vi "Read Config Unitest.vi"(8 "error in (no error)":errorcluster, 11 "main ref":T1) -> (0 "error out":errorcluster)   [LabVIEW 2025]
uses:
  controls/LAB-IQ UI Data.ctl
  Config file  FGV Unitest enum.ctl
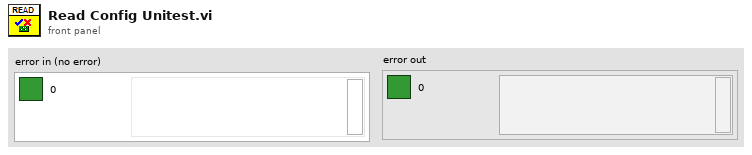
[diagram p1: front panel]
types:
  T1 = typedef "LAB-IQ UI Data.ctl" = cluster{"Main Home Screen":cluster{"GUI":refnum<vi>, "Platform Settings":refnum<vi>, "Configure":refnum<vi>, "Home":refnum<vi>, "EXIT":refnum<vi>, "service 2":refnum<vi>, "MainPage":refnum<vi>, "Analysis":refnum<vi>}, "Platform Settings":cluster{"mm/s  Surge":refnum<vi>, "Update Surge Speed":refnum<vi>, "Drive Error":refnum<vi>, "Disable Axis Jog Soft Limits":refnum<vi>, "mm/s  Sway":refnum<vi>, "Sway and Surge COM Status":refnum<vi>, "Heave COM Status":refnum<vi>, "Enable Platform":refnum<vi>, "Surge Forward Main":refnum<vi>, "Sway Right Main":refnum<vi>, "Sway Left Main":refnum<vi>, "Heave Down Main":refnum<vi>, "Heave Up main":refnum<vi>, "Update Sway Speed":refnum<vi>, "Update Heave Speed":refnum<vi>, "mm/s Heave":refnum<vi>, "mm/sec":refnum<vi>, "mm":refnum<vi>, "Surge Backward Main":refnum<vi>}, "Analysis Screen":cluster{"Analysis Home":refnum<vi>, "Surface Analysis":refnum<vi>, "Imaging":refnum<vi>, "Image Analysis":refnum<vi>, "Post Analysis":refnum<vi>}, "Config Screen":cluster{"Select Load Head":refnum<vi>, "Notes :":refnum<vi>, "FILE":refnum<vi>, "Sample ID :":refnum<vi>, "Operator ID :":refnum<vi>, "Operator Name :":refnum<vi>, "Auto":refnum<vi>}, "Motion Module":cluster{"zNL":refnum<vi>, "NL disp":refnum<vi>, "Rotary Tab":refnum<vi>, "Motion Direction:  3":refnum<vi>, "E.Velocity 2":refnum<vi>, "e.v/ssr 2":refnum<vi>, "Enter Fixed E.Velocity 2":refnum<vi>, "Enter Final SRR 2":refnum<vi>, "Enter initial SRR 2":refnum<vi>, "Enter Fixed SRR 2":refnum<vi>, "Enter the Final E.Velocity (m/s) 2":refnum<vi>, "Enter initial E.Velocity (m/s) 2":refnum<vi>, "Final Speed (RPM) 3":refnum<vi>, "Initial Speed (RPM) 2":refnum<vi>, "Enter the Final Velocity (m/s) 3":refnum<vi>, "Enter initial Velocity (m/s)  3":refnum<vi>, "Ramp Up 2":refnum<vi>, "TEST SELECTION":refnum<vi>, "SPEED SELECTION : ":refnum<vi>, "Angular Oscillation Set":refnum<vi>, "Traction":refnum<vi>, "Step Speed":refnum<vi>, "StepTable For Load-Speed":refnum<vi>, "StepTable For Speed":refnum<vi>, "Surge Forward MM":refnum<vi>, "Surge Backward MM":refnum<vi>, "M3 Image":refnum<vi>, "String 39":refnum<vi>, "Sway Left MM":refnum<vi>, "Sway Right MM":refnum<vi>, "Disable Axis Jog Soft Limits":refnum<vi>, "mm":refnum<vi>, "Heave Down MM":refnum<vi>, "Heave Up MM":refnum<vi>, "Wear Track Diameter (mm)":refnum<vi>, "Set WTD":refnum<vi>, "HomeScratch":refnum<vi>, "HomeRot":refnum<vi>, "PlaceModule":refnum<vi>, "Enter the Angle (Deg)":refnum<vi>, "Enter the Frequency (Hz)":refnum<vi>, "Motion Mode:":refnum<vi>, "LR Sway":refnum<vi>, "Rot Hor":refnum<vi>, "Scratch":refnum<vi>, "LR Cam":refnum<vi>, "MMBack":refnum<vi>, "MMNext":refnum<vi>, "Rot Ver":refnum<vi>, "Rotary Module Selection":refnum<vi>, "calculate rotary":refnum<vi>, "SPEED SELECTION : rotary":refnum<vi>, "Import 2":refnum<vi>, "Save 2":refnum<vi>, "File Path :  2":refnum<vi>, "String 45":refnum<vi>, "StepTable For Speed 3":refnum<vi>, "Enter the Speed(mm/sec)":refnum<vi>, "Enter the Speed(RPM)":refnum<vi>, "Enter Scratch Speed (mm/s):":refnum<vi>, "SwaySpeed Set":refnum<vi>, "Scartch Offset":refnum<vi>, "Motion type:":refnum<vi>, "HomeScratch 2":refnum<vi>, "Enter Scratch length (mm):":refnum<vi>, "Wear Track Diameter":refnum<vi>, "Rotary Speed Exced":refnum<vi>, "Scratch Mode":refnum<vi>, "No of Scratch":refnum<vi>}, "Environmental control":cluster{"Humidity  Status  3":refnum<vi>, "Low Temp  Status  2":refnum<vi>, "TK4 status 2":refnum<vi>, "Stage Temperature":refnum<vi>, "Sample Temperature":refnum<vi>, "Humidity (Amb)":refnum<vi>, "Clear List":refnum<vi>, "Add to list":refnum<vi>, "Wear":refnum<vi>, "Vibration":refnum<vi>, "Humidity (Chamber)":refnum<vi>, "Temperature (Chamber)":refnum<vi>, "ECR ":refnum<vi>, "Temperature (Amb)":refnum<vi>, "Microphone":refnum<vi>, "Acoustic Emission 3":refnum<vi>, "SNext":refnum<vi>, "APBack":refnum<vi>, "Enter the Temperature (°C):":refnum<vi>, "Enter the Stage \nTemperature (°C):":refnum<vi>, "Enter the Humidity (%Rh):":refnum<vi>, "Low Temp":refnum<vi>, "High Temp":refnum<vi>, "Humidity":refnum<vi>, "Sensors Picked":refnum<vi>}, "About Screen":cluster{"Password":refnum<vi>, "Home Service":refnum<vi>, "Advanced Setting":refnum<vi>, "About Tab":refnum<vi>, "ECR Port:":refnum<vi>, "Ramp Port:":refnum<vi>, "Installation/Replacement completed":refnum<vi>, "Loahead":refnum<vi>, "Heave and Surge COM Port:":refnum<vi>, "Sway COM Port:":refnum<vi>, "Temp Modbus:":refnum<vi>, "Humidity Port:":refnum<vi>, "Edit Gain Constants":refnum<vi>, "Save Gain Constants":refnum<vi>}, "Main Screen":cluster{"Main Screen Tab":refnum<vi>, "Angle and Frequency":refnum<vi>, "Stroke (mm)":refnum<vi>, "Angle (Deg)":refnum<vi>, "Main Speed Tab":refnum<vi>, "MTM MOTOR DISPLAY":refnum<vi>, "Disc Speed (m/sec)":refnum<vi>, "Ball Speed (m/sec)":refnum<vi>, "Disc Speed (RPM)":refnum<vi>, "Ball Speed (RPM)":refnum<vi>, "SPEED TAB":refnum<vi>, "Speed (m/sec)":refnum<vi>, "Set Speed (m/sec)":refnum<vi>, "Speed (RPM)":refnum<vi>, "Set Speed":refnum<vi>, "Time Tab":refnum<vi>, "Time ( HH:MM:SS ) 2":refnum<vi>, "Test Duration":refnum<vi>, "Test Duration 4":refnum<vi>, "TEST CYCLE":refnum<vi>, "TOTAL CYCLES":refnum<vi>, "Set Load (N)":refnum<vi>, "Temp Tabs":refnum<vi>, "Heater":refnum<vi>, "TK4 status":refnum<vi>, "ChamberTemp":refnum<vi>, "SetTmp":refnum<vi>, "Controller  Status":refnum<vi>, "ChamberTemp 2":refnum<vi>, "SetTmp 2":refnum<vi>, "Controller  Status 2":refnum<vi>, "ChamberTemp 3":refnum<vi>, "SetTmp 3":refnum<vi>, "Cooling":refnum<vi>, "Load Communication":refnum<vi>, "Ambient \nTemperature":refnum<vi>, "HumCOMStatus":refnum<vi>, "Ambient\n Humidity":refnum<vi>, "Freq (Hz)":refnum<vi>, "Load En":refnum<vi>, "NLt":refnum<vi>, "zNL 2":refnum<vi>, "Humidity On":refnum<vi>, "humidity disp":refnum<vi>, "Set Humidity":refnum<vi>, "NL disp 2":refnum<vi>, "Humidity On 2":refnum<vi>, "humidity disp 2":refnum<vi>, "Set Humidity 2":refnum<vi>, "NL disp 3":refnum<vi>, "AppLoadSeq scratch":refnum<vi>, "Stop Scratch":refnum<vi>, "ClrLog":refnum<vi>, "Trip Log":refnum<vi>, "STOP":refnum<vi>, "Start Test":refnum<vi>, "Test status":refnum<vi>, "AR Led":refnum<vi>, "Data":refnum<vi>, "Health":refnum<vi>, "Sway COM Status":refnum<vi>, "Heave COM Status":refnum<vi>, "Grp Tab":refnum<vi>, "Sub Graph":refnum<vi>, "SD (mm)":refnum<vi>, "Siliding distance Reset Graph":refnum<vi>, "SDGp":refnum<vi>, "Humidity Reset Graph":refnum<vi>, "HumrGp":refnum<vi>, "Acoustic Emission (mV)":refnum<vi>, "Aqucostic Reset Graph":refnum<vi>, "gACQUOS":refnum<vi>, "ECR RESET":refnum<vi>, "ECR":refnum<vi>, "Temperature Reset":refnum<vi>, "Acoustic Emission (mV) 2":refnum<vi>, "Aqucostic Reset Graph 2":refnum<vi>, "gACQUOS 2":refnum<vi>, "ECR RESET 2":refnum<vi>, "ECR 2":refnum<vi>, "Temperature Reset 2":refnum<vi>, "Temperature (deg c)":refnum<vi>, "Speed Reset Graph":refnum<vi>, "Speed Tab":refnum<vi>, "MTM DISC  SPEED":refnum<vi>, "MTM BALL SPEED":refnum<vi>, "speed mm/sec":refnum<vi>, "Hymidity":refnum<vi>, "Humidity Disable trip":refnum<vi>, "CoF Trip  2":refnum<vi>, "Depth Trip":refnum<vi>, "Weart Deapth":refnum<vi>, "Depth Reset Graph":refnum<vi>, "Weart":refnum<vi>, "Depthz":refnum<vi>, "Depth (µm)":refnum<vi>, "WearGp":refnum<vi>, "NL Trip 2":refnum<vi>, "Load pid":refnum<vi>, "Load Disable Trip":refnum<vi>, "Load Reset Graph":refnum<vi>, "NL Display 4":refnum<vi>, "Main Chart 3":refnum<vi>, "BACK":refnum<vi>, "Depth Trip 2":refnum<vi>, "COF TRIP ":refnum<vi>, "Friction Force (N)":refnum<vi>, "FF Reset Graph":refnum<vi>, "FF Disable Trip":refnum<vi>, "FF TRIP":refnum<vi>, "COF Disable Trip":refnum<vi>, "COF Reset Graph":refnum<vi>, "Start Test Temp":refnum<vi>, "zFF":refnum<vi>, "Friction Force (N) Graph":refnum<vi>, "Coefficient of Friction":refnum<vi>, "Scratch Start Test":refnum<vi>, "FF Tab":refnum<vi>, "Cyclic Friction Force (N)":refnum<vi>, "CZ FF":refnum<vi>, "Cyclic Friction Force (N) Graph":refnum<vi>, "Cyclic Coefficient of Friction":refnum<vi>, "Cyclic FF TRIP":refnum<vi>, "Cyclic FF Disable Trip":refnum<vi>, "cyclic COF Disable Trip":refnum<vi>, "cyclic COF TRIP":refnum<vi>, "cyclic COF Reset Graph":refnum<vi>, "Cyclic FF Reset Graph":refnum<vi>, "Test Trip":refnum<vi>, "Multi Scratch Pass":refnum<vi>}, "Loading":cluster{"Indentation":refnum<vi>, "Reference Sample":refnum<vi>, "Load Cell Communication Slide":refnum<vi>, "com 3":refnum<vi>, "com":refnum<vi>, "DecaForce COM Status":refnum<vi>, "Update":refnum<vi>, "Clear 3":refnum<vi>, "seq":refnum<vi>, "Stribeck table":refnum<vi>, "Stribeck Table  For loading":refnum<vi>, "Loading Mode":refnum<vi>, "Enter the Final Load (N)":refnum<vi>, "Enter the CoF Trip":refnum<vi>, "Enter the Friction Force Trip":refnum<vi>, "Enter the Normal load Trip":refnum<vi>, "Enter the Load  (N)":refnum<vi>, "KiloForce":refnum<vi>, "DecaForce ":refnum<vi>, "MicroForce":refnum<vi>, "LHBack":refnum<vi>, "LHNext":refnum<vi>, "Enter the Loading Rate (N/min)":refnum<vi>, "Message":refnum<vi>, "Warning 2":refnum<vi>, "SSP 0.75":refnum<vi>, "SSP 0.5":refnum<vi>, "SSP 0.3":refnum<vi>, "Warning":refnum<vi>, "gui GIF":refnum<vi>, "Communication is established":refnum<vi>, "AppLoad 4":refnum<vi>, "Multipoint":refnum<vi>, "Load Selection":refnum<vi>}, "PID":cluster{"Ramp MulFac":refnum<vi>, "pulses LoadDiffRamp(2..10)":refnum<vi>, "PulseControlRamp(diff<=3N)":refnum<vi>, "SetLoadDeadband(%) Load(0-10N)":refnum<vi>, "PID gains out delay (microForce)":refnum<vi>, "Ramp":refnum<vi>, "Gain 2":refnum<vi>, "pulses LoadDiff(2..10)":refnum<vi>, "pulses LoadDiff(11..50)":refnum<vi>, "PulseControl(diff<=3N)":refnum<vi>, "SetLoadDeadband(%)  2":refnum<vi>, "Dummy Run":refnum<vi>, "Vertical load (N)":refnum<vi>, "AutoTune":refnum<vi>, "Offset 3 ":refnum<vi>, "apply load":refnum<vi>, "Offset  3":refnum<vi>, "apply load 2":refnum<vi>, "Enter ByPass Load":refnum<vi>, "reinit 3":refnum<vi>, "output range delay":refnum<vi>, "PID gains out delay":refnum<vi>, "Bypass Load":refnum<vi>, "pulsesSent":refnum<vi>, "pulses ":refnum<vi>, "actpid":refnum<vi>, "gFF Rot":refnum<vi>, "pulses LoadDiff(21..1000)":refnum<vi>, "Delay":refnum<vi>, "deadband":refnum<vi>}, "Config Parameters":cluster{"Tab Control 3":refnum<vi>, "Tab Control 19":refnum<vi>, "SAMPLES":refnum<vi>, "Re-initilaize":refnum<vi>, "Filter ON/OFF":refnum<vi>, "TracHomeSurgeOffsetCounts 10MM":refnum<vi>, "TracHomeSwayOffsetCounts 10MM":refnum<vi>, "Acoustic Emission:":refnum<vi>, "Apply Filter (FF)":refnum<vi>, "Filter% 2":refnum<vi>, "Apply Filter (Load)":refnum<vi>, "Filter% ":refnum<vi>, "Sway distance (mm)":refnum<vi>, "Surge distance (mm)":refnum<vi>, "DataSavingLoopDelay(ms)":refnum<vi>, "SAVE 2":refnum<vi>, "Enter Distance":refnum<vi>, "Sway Counts:":refnum<vi>, "Distance (mm): 3":refnum<vi>, "Surge Counts:":refnum<vi>, "Distance (mm): 2":refnum<vi>, "Distance (mm):":refnum<vi>, "Heave Counts:":refnum<vi>, "LRMHomeSurgeOffsetCounts":refnum<vi>, "LRMHomeSwayOffsetCounts":refnum<vi>, "TracHomeSurgeOffsetCounts 20MM":refnum<vi>, "TracHomeSwayOffsetCounts 20MM":refnum<vi>, "RotHomeSwayOffsetCounts":refnum<vi>, "RotHomeSurgeOffsetCounts":refnum<vi>, "Heave distance":refnum<vi>, "Zmm":refnum<vi>, "Heave Pulses/mm":refnum<vi>, "Surge Pulses/mm":refnum<vi>, "Sway Pulses/mm":refnum<vi>, "Heave Pitch":refnum<vi>, "Surge Pitch":refnum<vi>, "Sway Pitch":refnum<vi>, "Heave PPR":refnum<vi>, "Surge PPR":refnum<vi>, "Sway PPR":refnum<vi>, "Tab Control 5":refnum<vi>, "Tab Control 14":refnum<vi>, "Tab Control 26":refnum<vi>, "AE":refnum<vi>, "Heave Loop Delay":refnum<vi>, "Heave PID Speed":refnum<vi>, "Surge Jog Speed":refnum<vi>, "Heave Jog Speed":refnum<vi>, "Sway Loop Delay":refnum<vi>, "Sway PID Speed":refnum<vi>, "Sway Jog Speed":refnum<vi>}, "Loading Com Port":cluster{"ClearAll":refnum<vi>, "Mz(Nm)":refnum<vi>, "My(Nm)":refnum<vi>, "Mx(Nm)":refnum<vi>, "Save Dwell":refnum<vi>, "Mx ":refnum<vi>, "My ":refnum<vi>, "Mz":refnum<vi>, "Fx(N)":refnum<vi>, "Fy(N)":refnum<vi>, "Fz(N)":refnum<vi>, "ZeroAll":refnum<vi>, "Acq Delay (ms)":refnum<vi>, "Burst Delay (ms)":refnum<vi>, "model":refnum<vi>, "SN":refnum<vi>, "FFx(N)":refnum<vi>, "Sensor IP":refnum<vi>, "Port":refnum<vi>, "FFy(N)":refnum<vi>, "Load(N)":refnum<vi>, "delete Handle":refnum<vi>, "Create Handle":refnum<vi>, "ft_data":refnum<vi>, "ft_range":refnum<vi>, "ft_data 2":refnum<vi>, "stop 6":refnum<vi>, "running_flag":refnum<vi>, "ft_udp_handle":refnum<vi>, "get-data-return":refnum<vi>, "get-range-return":refnum<vi>, "zero-return":refnum<vi>, "filter-return":refnum<vi>, "initial-return":refnum<vi>, "deleteHandle-result":refnum<vi>, "Load Cell Temp":refnum<vi>}, "Heave AND Surge":cluster{"SURGE POSE":refnum<vi>, "error out Read":refnum<vi>, "HEAVE POSE":refnum<vi>, "State":refnum<vi>, "Homed":refnum<vi>, "Sequence ID":refnum<vi>, "error out Write":refnum<vi>, "faultCode":refnum<vi>, "Ack ID":refnum<vi>, "SPEED":refnum<vi>, "Distance":refnum<vi>, "Mode Command":refnum<vi>, "Heave and Surge Read":refnum<vi>, "Read Heave Temp":refnum<vi>, "Spare 15":refnum<vi>, "Spare 14":refnum<vi>, "Spare 13":refnum<vi>, "Spare 12":refnum<vi>, "Spare 11":refnum<vi>, "Spare 10":refnum<vi>, "Spare 9":refnum<vi>, "Spare 8":refnum<vi>, "Spare 7":refnum<vi>, "Spare 6":refnum<vi>, "Spare 5":refnum<vi>, "Spare 4":refnum<vi>, "Spare 2":refnum<vi>, "Spare 1":refnum<vi>, "Node Id":refnum<vi>, "Spare 3":refnum<vi>, "SPARE 4":refnum<vi>, "SPARE 3":refnum<vi>, "SPARE 2":refnum<vi>, "SPARE 1":refnum<vi>, "fwMajor":refnum<vi>, "fwMinor":refnum<vi>, "Manual Write":refnum<vi>, "Heave and Surge Write":refnum<vi>}, "New PID LOGIC":cluster{"Fine Tune Zone":refnum<vi>, "PID SDelay":refnum<vi>, "Max_pos_limit":refnum<vi>, "Min_pos_limit":refnum<vi>, "i_limit":refnum<vi>, "pct_scale":refnum<vi>, "Deadband":refnum<vi>, "Kd":refnum<vi>, "Ki":refnum<vi>, "Kp":refnum<vi>, "Current Position":refnum<vi>, "Set Load":refnum<vi>, "Current Load":refnum<vi>, "Pulse delta":refnum<vi>, "Init Step":refnum<vi>, "Max Step Linit":refnum<vi>}, "SWAY ":cluster{"fwMajor":refnum<vi>, "Homed":refnum<vi>, "Rotary POSE":refnum<vi>, "State":refnum<vi>, "SWAY POSE":refnum<vi>, "Ack ID":refnum<vi>, "faultCode":refnum<vi>, "Node Id":refnum<vi>, "fwMinor":refnum<vi>, "Spare 6":refnum<vi>, "Spare 5":refnum<vi>, "Spare 4":refnum<vi>, "Spare 3":refnum<vi>, "Spare 2":refnum<vi>, "Spare 1":refnum<vi>, "Spare 7":refnum<vi>, "SPARE  5":refnum<vi>, "error out Write  SWAY ":refnum<vi>, "error out Read SWAY ":refnum<vi>, "Manual Write SWAY ":refnum<vi>, "SWAY WRITE":refnum<vi>, "SPARE  4":refnum<vi>, "SPARE  3":refnum<vi>, "SPARE 2":refnum<vi>, "SPARE 1":refnum<vi>, "Spare 15":refnum<vi>, "Spare 14":refnum<vi>, "Spare 13":refnum<vi>, "Spare 12":refnum<vi>, "Spare 11":refnum<vi>, "Spare 9":refnum<vi>, "Spare 8":refnum<vi>, "SPEED":refnum<vi>, "Distance":refnum<vi>, "Mode Command":refnum<vi>, "Sequence ID":refnum<vi>, "SWAY READ":refnum<vi>, "Spare 10":refnum<vi>, "Read SWAY Temp":refnum<vi>}, "Analysis Screen":cluster{"Analysis Home":refnum<vi>, "Refresh 2":refnum<vi>, "MEAN 4":refnum<vi>, "SD 4":refnum<vi>, "VARIANCE 4":refnum<vi>, "MEAN  3":refnum<vi>, "SD  3":refnum<vi>, "VARIANCE  3":refnum<vi>, "MEAN 2":refnum<vi>, "SD  2":refnum<vi>, "VARIANCE 2":refnum<vi>, "MEAN":refnum<vi>, "SD":refnum<vi>, "VARIANCE":refnum<vi>, "File 4 Discription":refnum<vi>, "OPEN 4":refnum<vi>, "File Name 4":refnum<vi>, "OPEN 3":refnum<vi>, "File 3 Discription":refnum<vi>, "File Name 3":refnum<vi>, "Y-AXIS":refnum<vi>, "X-AXIS":refnum<vi>, "XY Graph":refnum<vi>, "File Name 2":refnum<vi>, "File Name 1":refnum<vi>, "OPEN 2":refnum<vi>, "OPEN 1":refnum<vi>, "File 1 Discription ":refnum<vi>, "File 2 Discription":refnum<vi>}}
  T2 = typedef "Config file  FGV Unitest enum.ctl" = enum16{"OPEN", "READ", "WRITE", "CLOSE"}
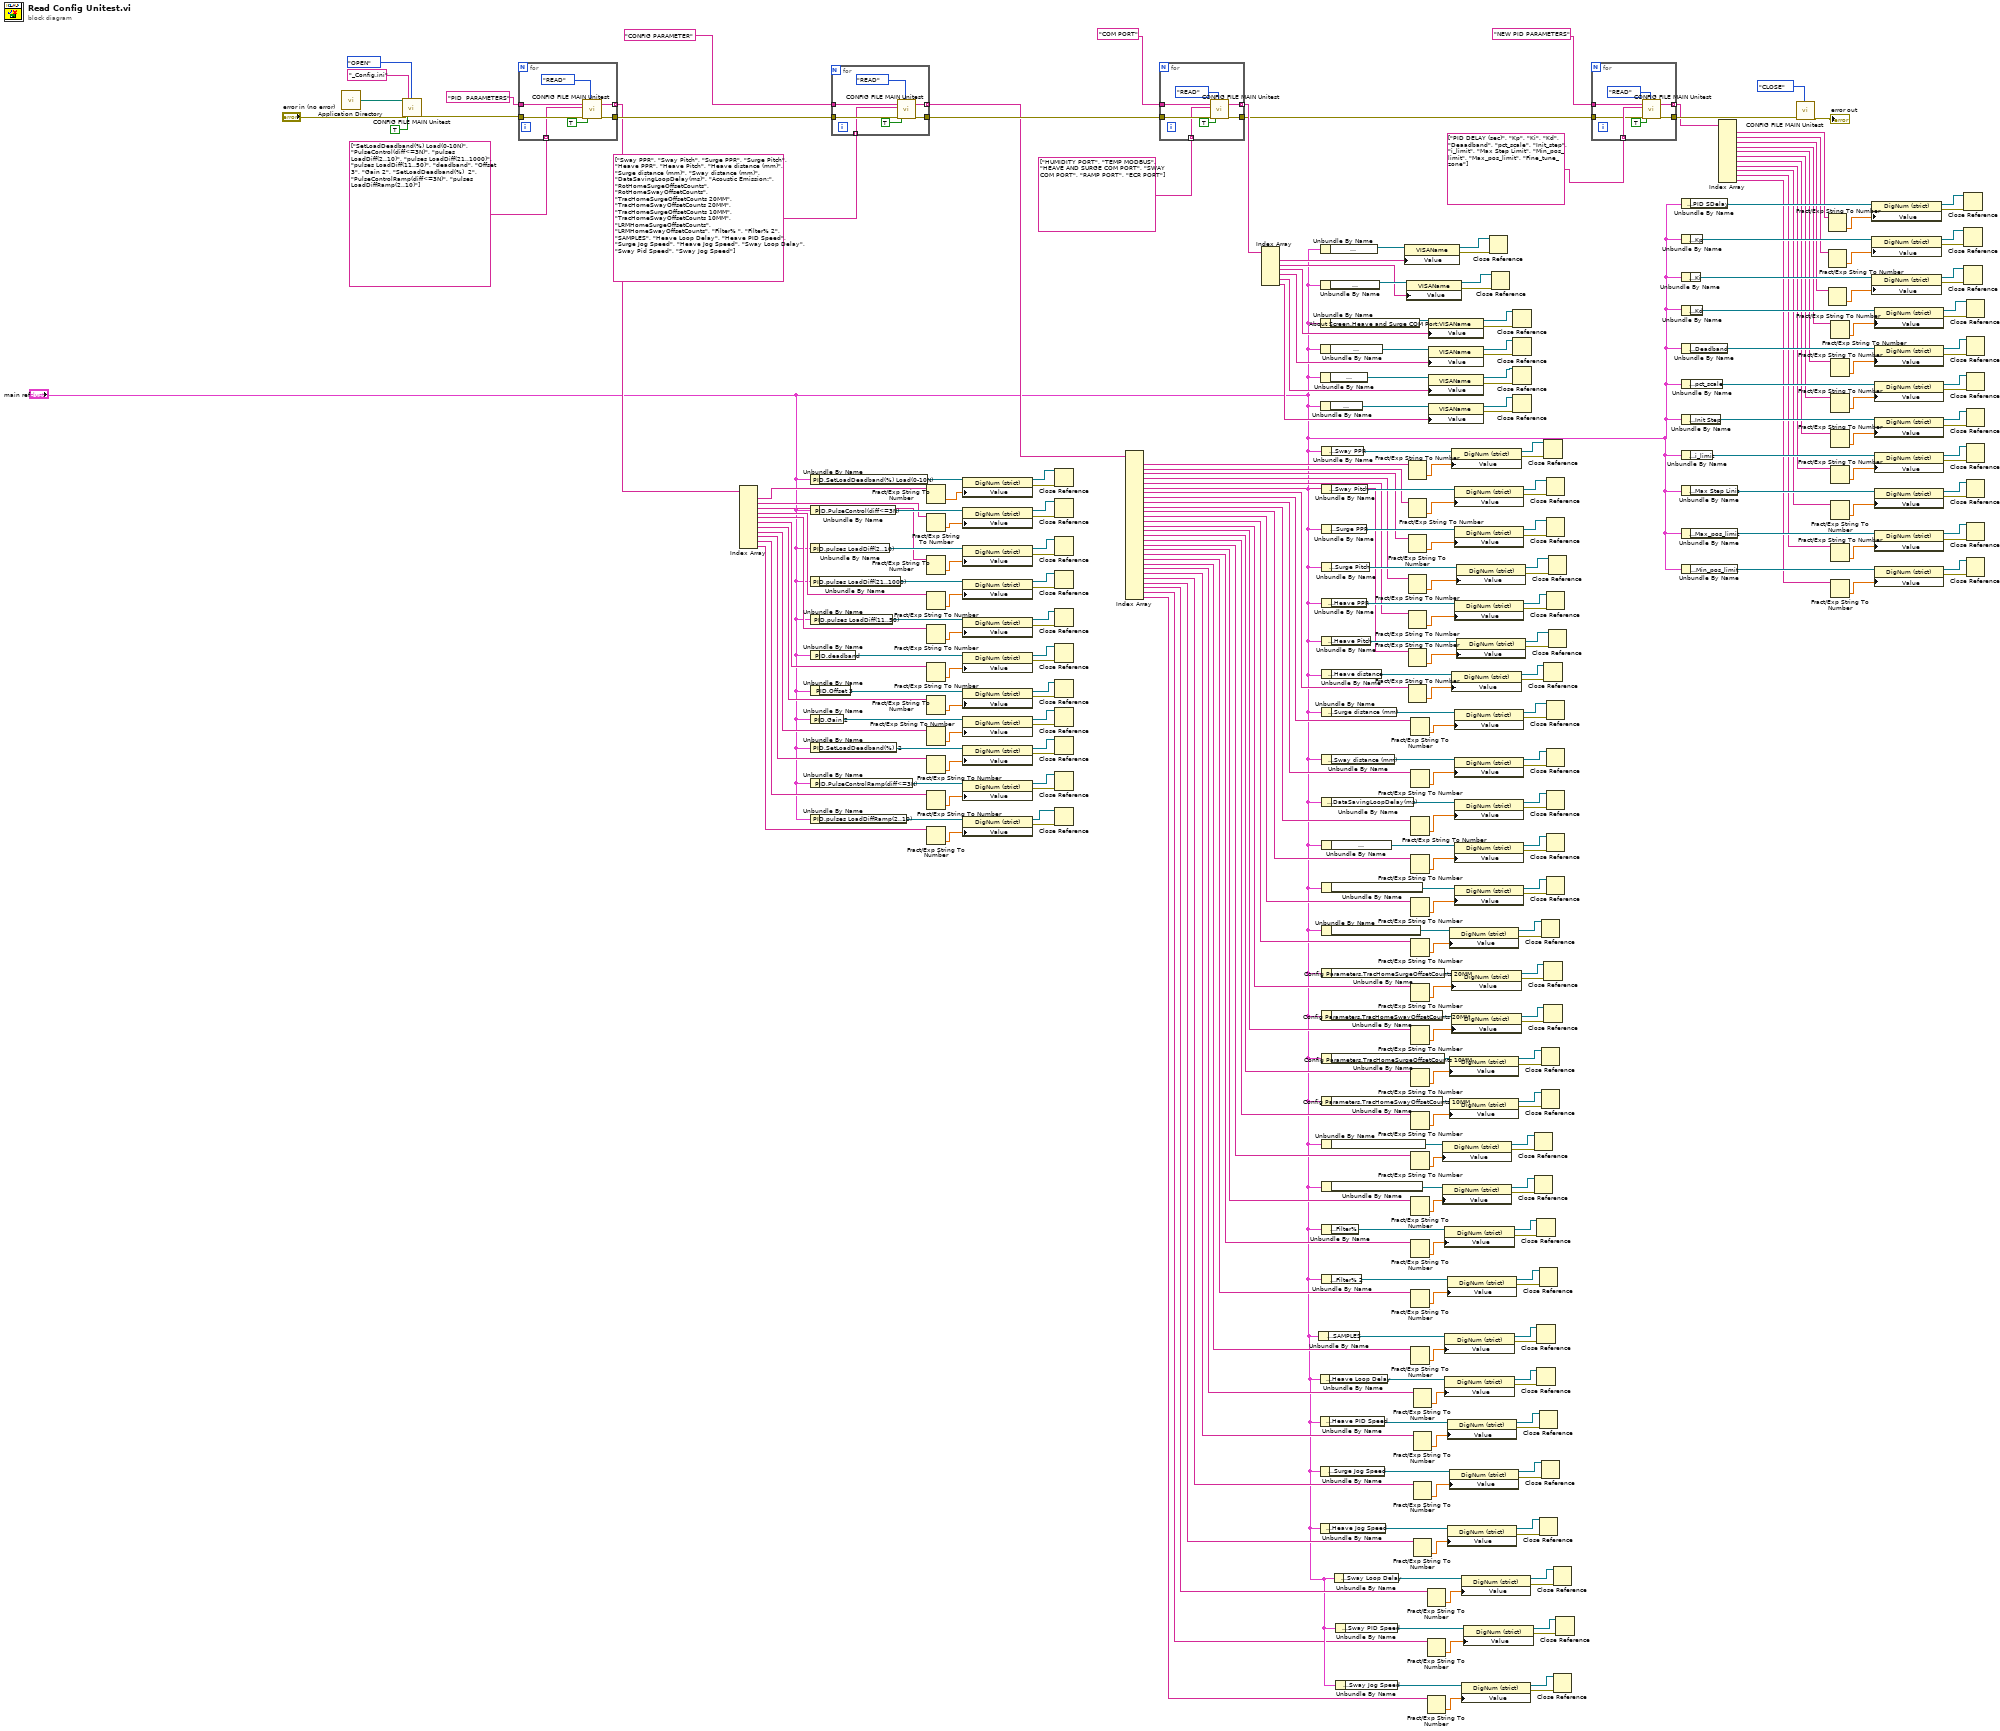
[diagram p0: block diagram]
diagram:
  n1 = call <vilib>:"Application Directory.vi"() -> ("Application Directory"=w300:path)
  n2 = call "CONFIG FILE MAIN Unitest.vi"("File Path"=w300, "error in"="error in (no error)", "file name"="_Config.ini", "PARAMETER/CONFIG"=TRUE, "Config Enum"=Config_file__FGV_Unitest_enum."OPEN") -> ("error out"=w299:errorcluster)  [unwired: 13 in, 1 out]
  n3 = for {
    tunnel: w299 -> [w311]
    tunnel: "PID  PARAMETERS" ("WRITE /READ SECTION") -> [w310]
    tunnel: string[] ["SetLoadDeadband(%) Load(0-10N)", "PulseControl(diff<=3N)", "pulses LoadDiff(2..10)", "pulses LoadDiff(21..1000)", "pulses LoadDiff(11..50)", "deadband", "Offset  3", "Gain 2", "SetLoadDeadband(%)  2", "PulseControlRamp(diff<=3N)", "pulses LoadDiffRamp(2..10)"] -> [w306] mode=indexing
    tunnel: [w309] -> w296
    tunnel: [w305] -> w109 mode=indexing
    n4 = call "CONFIG FILE MAIN Unitest.vi"("WRITE /READ SECTION"=w310, "READ KEY"=w306, "error in"=w311, "PARAMETER/CONFIG"=TRUE, "Config Enum"=Config_file__FGV_Unitest_enum."READ") -> ("READ VALUE"=w305:string, "error out"=w309:errorcluster)  [unwired: 13 in]
  }
  n5 = Index Array(array=w109) -> (element #1=w108:string, element #2=w107:string, element #3=w106:string, element #4=w105:string, element #5=w104:string, element #6=w103:string, element #7=w102:string, element #8=w101:string, element #9=w100:string, element #10=w99:string, element #11=w98:string)  [unwired: 11 in]
  n6 = Unbundle By Name("main ref") -> ("PID.SetLoadDeadband(%) Load(0-10N)"=w290:refnum<vi>)
  n7 = Unbundle By Name("main ref") -> ("PID.PulseControl(diff<=3N)"=w285:refnum<vi>)
  n8 = Unbundle By Name("main ref") -> ("PID.pulses LoadDiff(2..10)"=w284:refnum<vi>)
  n9 = Unbundle By Name("main ref") -> ("PID.pulses LoadDiff(21..1000)"=w279:refnum<vi>)
  n10 = Unbundle By Name("main ref") -> ("PID.pulses LoadDiff(11..50)"=w278:refnum<vi>)
  n11 = Unbundle By Name("main ref") -> ("PID.deadband"=w273:refnum<vi>)
  n12 = Unbundle By Name("main ref") -> ("PID.Offset 3"=w272:refnum<vi>)
  n13 = Unbundle By Name("main ref") -> ("PID.Gain 2"=w267:refnum<vi>)
  n14 = Unbundle By Name("main ref") -> ("PID.SetLoadDeadband(%)  2"=w266:refnum<vi>)
  n15 = Unbundle By Name("main ref") -> ("PID.PulseControlRamp(diff<=3N)"=w262:refnum<vi>)
  n16 = Unbundle By Name("main ref") -> ("PID.pulses LoadDiffRamp(2..10)"=w260:refnum<vi>)
  n17 = for {
    tunnel: w296 -> [w318]
    tunnel: "CONFIG PARAMETER" ("WRITE /READ SECTION") -> [w317]
    tunnel: [w316] -> w294
    tunnel: string[] ["Sway PPR", "Sway Pitch", "Surge PPR", "Surge Pitch", "Heave PPR", "Heave Pitch", "Heave distance (mm)", "Surge distance (mm)", "Sway distance (mm)", "DataSavingLoopDelay(ms)", "Acoustic Emission:", "RotHomeSurgeOffsetCounts", "RotHomeSwayOffsetCounts", "TracHomeSurgeOffsetCounts 20MM", "TracHomeSwayOffsetCounts 20MM", "TracHomeSurgeOffsetCounts 10MM", "TracHomeSwayOffsetCounts 10MM", "LRMHomeSurgeOffsetCounts", "LRMHomeSwayOffsetCounts", "Filter% ", "Filter% 2", "SAMPLES", "Heave Loop Delay", "Heave PID Speed", "Surge Jog Speed", "Heave Jog Speed", "Sway Loop Delay", "Sway Pid Speed", "Sway Jog Speed"] -> [w313] mode=indexing
    tunnel: [w312] -> w165 mode=indexing
    n18 = call "CONFIG FILE MAIN Unitest.vi"("WRITE /READ SECTION"=w317, "READ KEY"=w313, "error in"=w318, "PARAMETER/CONFIG"=TRUE, "Config Enum"=Config_file__FGV_Unitest_enum."READ") -> ("READ VALUE"=w312:string, "error out"=w316:errorcluster)  [unwired: 13 in]
  }
  n19 = Fract/Exp String To Number(string=w108) -> (number=w120:dbl)  [unwired: 3 in, 1 out]
  n20 = Fract/Exp String To Number(string=w107) -> (number=w119:dbl)  [unwired: 3 in, 1 out]
  n21 = Fract/Exp String To Number(string=w106) -> (number=w118:dbl)  [unwired: 3 in, 1 out]
  n22 = Fract/Exp String To Number(string=w105) -> (number=w117:dbl)  [unwired: 3 in, 1 out]
  n23 = Fract/Exp String To Number(string=w104) -> (number=w116:dbl)  [unwired: 3 in, 1 out]
  n24 = Fract/Exp String To Number(string=w103) -> (number=w115:dbl)  [unwired: 3 in, 1 out]
  n25 = Fract/Exp String To Number(string=w102) -> (number=w114:dbl)  [unwired: 3 in, 1 out]
  n26 = Fract/Exp String To Number(string=w101) -> (number=w113:dbl)  [unwired: 3 in, 1 out]
  n27 = Fract/Exp String To Number(string=w100) -> (number=w112:dbl)  [unwired: 3 in, 1 out]
  n28 = Fract/Exp String To Number(string=w99) -> (number=w111:dbl)  [unwired: 3 in, 1 out]
  n29 = Fract/Exp String To Number(string=w98) -> (number=w110:dbl)  [unwired: 3 in, 1 out]
  n30 = property class="DigNum (strict)"(reference=w290, "Value"=w120) -> (reference out=w288:refnum<vi>, error out=w289:errorcluster)  [unwired: 1 in]
  n31 = property class="DigNum (strict)"(reference=w285, "Value"=w119) -> (reference out=w287:refnum<vi>, error out=w286:errorcluster)  [unwired: 1 in]
  n32 = property class="DigNum (strict)"(reference=w284, "Value"=w118) -> (reference out=w282:refnum<vi>, error out=w283:errorcluster)  [unwired: 1 in]
  n33 = property class="DigNum (strict)"(reference=w279, "Value"=w117) -> (reference out=w281:refnum<vi>, error out=w280:errorcluster)  [unwired: 1 in]
  n34 = property class="DigNum (strict)"(reference=w278, "Value"=w116) -> (reference out=w276:refnum<vi>, error out=w277:errorcluster)  [unwired: 1 in]
  n35 = property class="DigNum (strict)"(reference=w273, "Value"=w115) -> (reference out=w275:refnum<vi>, error out=w274:errorcluster)  [unwired: 1 in]
  n36 = property class="DigNum (strict)"(reference=w272, "Value"=w114) -> (reference out=w270:refnum<vi>, error out=w271:errorcluster)  [unwired: 1 in]
  n37 = property class="DigNum (strict)"(reference=w267, "Value"=w113) -> (reference out=w269:refnum<vi>, error out=w268:errorcluster)  [unwired: 1 in]
  n38 = property class="DigNum (strict)"(reference=w266, "Value"=w112) -> (reference out=w264:refnum<vi>, error out=w265:errorcluster)  [unwired: 1 in]
  n39 = property class="DigNum (strict)"(reference=w262, "Value"=w111) -> (reference out=w261:refnum<vi>, error out=w263:errorcluster)  [unwired: 1 in]
  n40 = property class="DigNum (strict)"(reference=w260, "Value"=w110) -> (reference out=w258:refnum<vi>, error out=w259:errorcluster)  [unwired: 1 in]
  n41 = Close Reference(reference=w288, error in (no error)=w289) -> ()  [unwired: 1 out]
  n42 = Close Reference(reference=w287, error in (no error)=w286) -> ()  [unwired: 1 out]
  n43 = Close Reference(reference=w282, error in (no error)=w283) -> ()  [unwired: 1 out]
  n44 = Close Reference(reference=w281, error in (no error)=w280) -> ()  [unwired: 1 out]
  n45 = Close Reference(reference=w276, error in (no error)=w277) -> ()  [unwired: 1 out]
  n46 = Close Reference(reference=w275, error in (no error)=w274) -> ()  [unwired: 1 out]
  n47 = Close Reference(reference=w270, error in (no error)=w271) -> ()  [unwired: 1 out]
  n48 = Close Reference(reference=w269, error in (no error)=w268) -> ()  [unwired: 1 out]
  n49 = Close Reference(reference=w264, error in (no error)=w265) -> ()  [unwired: 1 out]
  n50 = Close Reference(reference=w261, error in (no error)=w263) -> ()  [unwired: 1 out]
  n51 = Close Reference(reference=w258, error in (no error)=w259) -> ()  [unwired: 1 out]
  n52 = Index Array(array=w165) -> (element #1=w164:string, element #2=w163:string, element #3=w162:string, element #4=w161:string, element #5=w160:string, element #6=w159:string, element #7=w158:string, element #8=w157:string, element #9=w156:string, element #10=w155:string, element #11=w154:string, element #12=w153:string, element #13=w152:string, element #14=w151:string, element #15=w150:string, element #16=w149:string, element #17=w148:string, element #18=w147:string, element #19=w146:string, element #20=w145:string, element #21=w144:string, element #22=w143:string, element #23=w81:string, element #24=w80:string, element #25=w79:string, element #26=w78:string, element #27=w4:string, element #28=w2:string, element #29=w1:string)  [unwired: 29 in]
  n53 = for {
    tunnel: w294 -> [w325]
    tunnel: "COM PORT" ("WRITE /READ SECTION") -> [w324]
    tunnel: [w323] -> w76
    tunnel: string[] ["HUMIDITY PORT", "TEMP MODBUS", "HEAVE AND SURGE COM PORT", "SWAY COM PORT", "RAMP PORT", "ECR PORT"] -> [w320] mode=indexing
    tunnel: [w319] -> w172 mode=indexing
    n54 = call "CONFIG FILE MAIN Unitest.vi"("WRITE /READ SECTION"=w324, "READ KEY"=w320, "error in"=w325, "PARAMETER/CONFIG"=TRUE, "Config Enum"=Config_file__FGV_Unitest_enum."READ") -> ("READ VALUE"=w319:string, "error out"=w323:errorcluster)  [unwired: 13 in]
  }
  n55 = Index Array(array=w172) -> (element #1=w171:string, element #2=w170:string, element #3=w169:string, element #4=w168:string, element #5=w167:string, element #6=w166:string)  [unwired: 6 in]
  n56 = Unbundle By Name("main ref") -> ("Config Parameters.SAMPLES"=w196:refnum<vi>)
  n57 = Unbundle By Name("main ref") -> ("Config Parameters.Heave Loop Delay"=w84:refnum<vi>)
  n58 = Unbundle By Name("main ref") -> ("Config Parameters.Heave PID Speed"=w85:refnum<vi>)
  n59 = Unbundle By Name("main ref") -> ("Config Parameters.Surge Jog Speed"=w89:refnum<vi>)
  n60 = Unbundle By Name("main ref") -> ("Config Parameters.Heave Jog Speed"=w90:refnum<vi>)
  n61 = Unbundle By Name("main ref") -> ("About Screen.Humidity Port:"=w190:refnum<vi>)
  n62 = Unbundle By Name("main ref") -> ("About Screen.Temp Modbus:"=w185:refnum<vi>)
  n63 = Unbundle By Name("main ref") -> ("About Screen.Heave and Surge COM Port:"=w184:refnum<vi>)
  n64 = Unbundle By Name("main ref") -> ("About Screen.Sway COM Port:"=w180:refnum<vi>)
  n65 = Unbundle By Name("main ref") -> ("About Screen.Ramp Port:"=w179:refnum<vi>)
  n66 = Unbundle By Name("main ref") -> ("About Screen.ECR Port:"=w176:refnum<vi>)
  n67 = Unbundle By Name("main ref") -> ("Config Parameters.Sway PPR"=w257:refnum<vi>)
  n68 = Unbundle By Name("main ref") -> ("Config Parameters.Sway Pitch"=w252:refnum<vi>)
  n69 = Unbundle By Name("main ref") -> ("Config Parameters.Surge PPR"=w246:refnum<vi>)
  n70 = Unbundle By Name("main ref") -> ("Config Parameters.Surge Pitch"=w251:refnum<vi>)
  n71 = Unbundle By Name("main ref") -> ("Config Parameters.Heave PPR"=w245:refnum<vi>)
  n72 = Unbundle By Name("main ref") -> ("Config Parameters.Heave Pitch"=w241:refnum<vi>)
  n73 = Unbundle By Name("main ref") -> ("Config Parameters.Heave distance"=w235:refnum<vi>)
  n74 = Unbundle By Name("main ref") -> ("Config Parameters.Surge distance (mm)"=w239:refnum<vi>)
  n75 = Unbundle By Name("main ref") -> ("Config Parameters.Sway distance (mm)"=w233:refnum<vi>)
  n76 = Unbundle By Name("main ref") -> ("Config Parameters.DataSavingLoopDelay(ms)"=w230:refnum<vi>)
  n77 = Unbundle By Name("main ref") -> ("Config Parameters.Acoustic Emission:"=w227:refnum<vi>)
  n78 = Unbundle By Name("main ref") -> ("Config Parameters.RotHomeSurgeOffsetCounts"=w224:refnum<vi>)
  n79 = Unbundle By Name("main ref") -> ("Config Parameters.RotHomeSwayOffsetCounts"=w221:refnum<vi>)
  n80 = Unbundle By Name("main ref") -> ("Config Parameters.TracHomeSurgeOffsetCounts 20MM"=w218:refnum<vi>)
  n81 = Unbundle By Name("main ref") -> ("Config Parameters.TracHomeSwayOffsetCounts 20MM"=w215:refnum<vi>)
  n82 = Unbundle By Name("main ref") -> ("Config Parameters.TracHomeSurgeOffsetCounts 10MM"=w211:refnum<vi>)
  n83 = Unbundle By Name("main ref") -> ("Config Parameters.TracHomeSwayOffsetCounts 10MM"=w214:refnum<vi>)
  n84 = Unbundle By Name("main ref") -> ("Config Parameters.LRMHomeSurgeOffsetCounts"=w205:refnum<vi>)
  n85 = Unbundle By Name("main ref") -> ("Config Parameters.LRMHomeSwayOffsetCounts"=w202:refnum<vi>)
  n86 = Unbundle By Name("main ref") -> ("Config Parameters.Filter%"=w201:refnum<vi>)
  n87 = Unbundle By Name("main ref") -> ("Config Parameters.Filter% 2"=w197:refnum<vi>)
  n88 = Unbundle By Name("main ref") -> ("Config Parameters.Sway Loop Delay"=w16:refnum<vi>)
  n89 = Unbundle By Name("main ref") -> ("Config Parameters.Sway PID Speed"=w12:refnum<vi>)
  n90 = Unbundle By Name("main ref") -> ("Config Parameters.Sway Jog Speed"=w11:refnum<vi>)
  n91 = property class="VISAName"(reference=w190, "Value"=w171) -> (reference out=w188:refnum<vi>, error out=w189:errorcluster)  [unwired: 1 in]
  n92 = property class="VISAName"(reference=w185, "Value"=w170) -> (reference out=w187:refnum<vi>, error out=w186:errorcluster)  [unwired: 1 in]
  n93 = Fract/Exp String To Number(string=w164) -> (number=w142:dbl)  [unwired: 3 in, 1 out]
  n94 = Fract/Exp String To Number(string=w163) -> (number=w141:dbl)  [unwired: 3 in, 1 out]
  n95 = Fract/Exp String To Number(string=w162) -> (number=w140:dbl)  [unwired: 3 in, 1 out]
  n96 = Fract/Exp String To Number(string=w161) -> (number=w139:dbl)  [unwired: 3 in, 1 out]
  n97 = Fract/Exp String To Number(string=w160) -> (number=w138:dbl)  [unwired: 3 in, 1 out]
  n98 = Fract/Exp String To Number(string=w159) -> (number=w137:dbl)  [unwired: 3 in, 1 out]
  n99 = Fract/Exp String To Number(string=w158) -> (number=w136:dbl)  [unwired: 3 in, 1 out]
  n100 = Fract/Exp String To Number(string=w157) -> (number=w135:dbl)  [unwired: 3 in, 1 out]
  n101 = Fract/Exp String To Number(string=w156) -> (number=w134:dbl)  [unwired: 3 in, 1 out]
  n102 = Fract/Exp String To Number(string=w155) -> (number=w133:dbl)  [unwired: 3 in, 1 out]
  n103 = Fract/Exp String To Number(string=w154) -> (number=w132:dbl)  [unwired: 3 in, 1 out]
  n104 = Fract/Exp String To Number(string=w153) -> (number=w131:dbl)  [unwired: 3 in, 1 out]
  n105 = Fract/Exp String To Number(string=w152) -> (number=w130:dbl)  [unwired: 3 in, 1 out]
  n106 = Fract/Exp String To Number(string=w151) -> (number=w129:dbl)  [unwired: 3 in, 1 out]
  n107 = Fract/Exp String To Number(string=w150) -> (number=w128:dbl)  [unwired: 3 in, 1 out]
  n108 = Fract/Exp String To Number(string=w149) -> (number=w127:dbl)  [unwired: 3 in, 1 out]
  n109 = Fract/Exp String To Number(string=w148) -> (number=w126:dbl)  [unwired: 3 in, 1 out]
  n110 = Fract/Exp String To Number(string=w147) -> (number=w125:dbl)  [unwired: 3 in, 1 out]
  n111 = Fract/Exp String To Number(string=w146) -> (number=w124:dbl)  [unwired: 3 in, 1 out]
  n112 = Fract/Exp String To Number(string=w145) -> (number=w123:dbl)  [unwired: 3 in, 1 out]
  n113 = Fract/Exp String To Number(string=w144) -> (number=w122:dbl)  [unwired: 3 in, 1 out]
  n114 = Fract/Exp String To Number(string=w143) -> (number=w121:dbl)  [unwired: 3 in, 1 out]
  n115 = Fract/Exp String To Number(string=w81) -> (number=w94:dbl)  [unwired: 3 in, 1 out]
  n116 = Fract/Exp String To Number(string=w80) -> (number=w95:dbl)  [unwired: 3 in, 1 out]
  n117 = Fract/Exp String To Number(string=w79) -> (number=w96:dbl)  [unwired: 3 in, 1 out]
  n118 = Fract/Exp String To Number(string=w78) -> (number=w97:dbl)  [unwired: 3 in, 1 out]
  n119 = Fract/Exp String To Number(string=w4) -> (number=w7:dbl)  [unwired: 3 in, 1 out]
  n120 = Fract/Exp String To Number(string=w2) -> (number=w6:dbl)  [unwired: 3 in, 1 out]
  n121 = Fract/Exp String To Number(string=w1) -> (number=w5:dbl)  [unwired: 3 in, 1 out]
  n122 = property class="VISAName"(reference=w184, "Value"=w169) -> (reference out=w182:refnum<vi>, error out=w183:errorcluster)  [unwired: 1 in]
  n123 = property class="VISAName"(reference=w180, "Value"=w168) -> (reference out=w175:refnum<vi>, error out=w181:errorcluster)  [unwired: 1 in]
  n124 = property class="VISAName"(reference=w179, "Value"=w167) -> (reference out=w174:refnum<vi>, error out=w178:errorcluster)  [unwired: 1 in]
  n125 = property class="VISAName"(reference=w176, "Value"=w166) -> (reference out=w173:refnum<vi>, error out=w177:errorcluster)  [unwired: 1 in]
  n126 = property class="DigNum (strict)"(reference=w205, "Value"=w125) -> (reference out=w206:refnum<vi>, error out=w204:errorcluster)  [unwired: 1 in]
  n127 = property class="DigNum (strict)"(reference=w202, "Value"=w124) -> (reference out=w207:refnum<vi>, error out=w203:errorcluster)  [unwired: 1 in]
  n128 = property class="DigNum (strict)"(reference=w201, "Value"=w123) -> (reference out=w199:refnum<vi>, error out=w200:errorcluster)  [unwired: 1 in]
  n129 = property class="DigNum (strict)"(reference=w196, "Value"=w121) -> (reference out=w194:refnum<vi>, error out=w195:errorcluster)  [unwired: 1 in]
  n130 = property class="DigNum (strict)"(reference=w84, "Value"=w94) -> (reference out=w82:refnum<vi>, error out=w83:errorcluster)  [unwired: 1 in]
  n131 = property class="DigNum (strict)"(reference=w197, "Value"=w122) -> (reference out=w193:refnum<vi>, error out=w198:errorcluster)  [unwired: 1 in]
  n132 = property class="DigNum (strict)"(reference=w85, "Value"=w95) -> (reference out=w87:refnum<vi>, error out=w86:errorcluster)  [unwired: 1 in]
  n133 = property class="DigNum (strict)"(reference=w90, "Value"=w97) -> (reference out=w92:refnum<vi>, error out=w91:errorcluster)  [unwired: 1 in]
  n134 = property class="DigNum (strict)"(reference=w221, "Value"=w130) -> (reference out=w220:refnum<vi>, error out=w222:errorcluster)  [unwired: 1 in]
  n135 = property class="DigNum (strict)"(reference=w211, "Value"=w127) -> (reference out=w209:refnum<vi>, error out=w212:errorcluster)  [unwired: 1 in]
  n136 = property class="DigNum (strict)"(reference=w214, "Value"=w126) -> (reference out=w208:refnum<vi>, error out=w213:errorcluster)  [unwired: 1 in]
  n137 = property class="DigNum (strict)"(reference=w89, "Value"=w96) -> (reference out=w93:refnum<vi>, error out=w88:errorcluster)  [unwired: 1 in]
  n138 = property class="DigNum (strict)"(reference=w257, "Value"=w142) -> (reference out=w255:refnum<vi>, error out=w256:errorcluster)  [unwired: 1 in]
  n139 = property class="DigNum (strict)"(reference=w235, "Value"=w136) -> (reference out=w192:refnum<vi>, error out=w236:errorcluster)  [unwired: 1 in]
  n140 = property class="DigNum (strict)"(reference=w218, "Value"=w129) -> (reference out=w219:refnum<vi>, error out=w217:errorcluster)  [unwired: 1 in]
  n141 = property class="DigNum (strict)"(reference=w215, "Value"=w128) -> (reference out=w210:refnum<vi>, error out=w216:errorcluster)  [unwired: 1 in]
  n142 = property class="DigNum (strict)"(reference=w252, "Value"=w141) -> (reference out=w254:refnum<vi>, error out=w253:errorcluster)  [unwired: 1 in]
  n143 = property class="DigNum (strict)"(reference=w246, "Value"=w140) -> (reference out=w248:refnum<vi>, error out=w247:errorcluster)  [unwired: 1 in]
  n144 = property class="DigNum (strict)"(reference=w245, "Value"=w138) -> (reference out=w240:refnum<vi>, error out=w244:errorcluster)  [unwired: 1 in]
  n145 = property class="DigNum (strict)"(reference=w239, "Value"=w135) -> (reference out=w237:refnum<vi>, error out=w238:errorcluster)  [unwired: 1 in]
  n146 = property class="DigNum (strict)"(reference=w233, "Value"=w134) -> (reference out=w232:refnum<vi>, error out=w234:errorcluster)  [unwired: 1 in]
  n147 = property class="DigNum (strict)"(reference=w230, "Value"=w133) -> (reference out=w231:refnum<vi>, error out=w229:errorcluster)  [unwired: 1 in]
  n148 = property class="DigNum (strict)"(reference=w227, "Value"=w132) -> (reference out=w226:refnum<vi>, error out=w228:errorcluster)  [unwired: 1 in]
  n149 = property class="DigNum (strict)"(reference=w224, "Value"=w131) -> (reference out=w225:refnum<vi>, error out=w223:errorcluster)  [unwired: 1 in]
  n150 = property class="DigNum (strict)"(reference=w251, "Value"=w139) -> (reference out=w249:refnum<vi>, error out=w250:errorcluster)  [unwired: 1 in]
  n151 = property class="DigNum (strict)"(reference=w241, "Value"=w137) -> (reference out=w243:refnum<vi>, error out=w242:errorcluster)  [unwired: 1 in]
  n152 = property class="DigNum (strict)"(reference=w16, "Value"=w7) -> (reference out=w14:refnum<vi>, error out=w15:errorcluster)  [unwired: 1 in]
  n153 = property class="DigNum (strict)"(reference=w11, "Value"=w5) -> (reference out=w9:refnum<vi>, error out=w10:errorcluster)  [unwired: 1 in]
  n154 = property class="DigNum (strict)"(reference=w12, "Value"=w6) -> (reference out=w8:refnum<vi>, error out=w13:errorcluster)  [unwired: 1 in]
  n155 = Close Reference(reference=w188, error in (no error)=w189) -> ()  [unwired: 1 out]
  n156 = Close Reference(reference=w187, error in (no error)=w186) -> ()  [unwired: 1 out]
  n157 = Close Reference(reference=w182, error in (no error)=w183) -> ()  [unwired: 1 out]
  n158 = Close Reference(reference=w175, error in (no error)=w181) -> ()  [unwired: 1 out]
  n159 = Close Reference(reference=w174, error in (no error)=w178) -> ()  [unwired: 1 out]
  n160 = Close Reference(reference=w173, error in (no error)=w177) -> ()  [unwired: 1 out]
  n161 = Close Reference(reference=w206, error in (no error)=w204) -> ()  [unwired: 1 out]
  n162 = Close Reference(reference=w207, error in (no error)=w203) -> ()  [unwired: 1 out]
  n163 = Close Reference(reference=w199, error in (no error)=w200) -> ()  [unwired: 1 out]
  n164 = Close Reference(reference=w194, error in (no error)=w195) -> ()  [unwired: 1 out]
  n165 = Close Reference(reference=w82, error in (no error)=w83) -> ()  [unwired: 1 out]
  n166 = Close Reference(reference=w193, error in (no error)=w198) -> ()  [unwired: 1 out]
  n167 = Close Reference(reference=w87, error in (no error)=w86) -> ()  [unwired: 1 out]
  n168 = Close Reference(reference=w92, error in (no error)=w91) -> ()  [unwired: 1 out]
  n169 = Close Reference(reference=w220, error in (no error)=w222) -> ()  [unwired: 1 out]
  n170 = Close Reference(reference=w209, error in (no error)=w212) -> ()  [unwired: 1 out]
  n171 = Close Reference(reference=w208, error in (no error)=w213) -> ()  [unwired: 1 out]
  n172 = Close Reference(reference=w93, error in (no error)=w88) -> ()  [unwired: 1 out]
  n173 = Close Reference(reference=w255, error in (no error)=w256) -> ()  [unwired: 1 out]
  n174 = Close Reference(reference=w192, error in (no error)=w236) -> ()  [unwired: 1 out]
  n175 = Close Reference(reference=w219, error in (no error)=w217) -> ()  [unwired: 1 out]
  n176 = Close Reference(reference=w210, error in (no error)=w216) -> ()  [unwired: 1 out]
  n177 = Close Reference(reference=w254, error in (no error)=w253) -> ()  [unwired: 1 out]
  n178 = Close Reference(reference=w248, error in (no error)=w247) -> ()  [unwired: 1 out]
  n179 = Close Reference(reference=w240, error in (no error)=w244) -> ()  [unwired: 1 out]
  n180 = Close Reference(reference=w237, error in (no error)=w238) -> ()  [unwired: 1 out]
  n181 = Close Reference(reference=w232, error in (no error)=w234) -> ()  [unwired: 1 out]
  n182 = Close Reference(reference=w231, error in (no error)=w229) -> ()  [unwired: 1 out]
  n183 = Close Reference(reference=w226, error in (no error)=w228) -> ()  [unwired: 1 out]
  n184 = Close Reference(reference=w225, error in (no error)=w223) -> ()  [unwired: 1 out]
  n185 = Close Reference(reference=w249, error in (no error)=w250) -> ()  [unwired: 1 out]
  n186 = Close Reference(reference=w243, error in (no error)=w242) -> ()  [unwired: 1 out]
  n187 = Close Reference(reference=w14, error in (no error)=w15) -> ()  [unwired: 1 out]
  n188 = Close Reference(reference=w9, error in (no error)=w10) -> ()  [unwired: 1 out]
  n189 = Close Reference(reference=w8, error in (no error)=w13) -> ()  [unwired: 1 out]
  n190 = for {
    tunnel: "NEW PID PARAMETERS" ("WRITE /READ SECTION") -> [w332]
    tunnel: [w331] -> w75
    tunnel: string[] ["PID DELAY (sec)", "Kp", "Ki", "Kd", "Deaadband", "pct_scale", "Init_step", "i_limit", "Max Step Limit", "Min_pos_limit", "Max_pos_limit", "Fine_tune_zone"] -> [w328] mode=indexing
    tunnel: [w327] -> w47 mode=indexing
    tunnel: w76 -> [w326]
    n191 = call "CONFIG FILE MAIN Unitest.vi"("WRITE /READ SECTION"=w332, "READ KEY"=w328, "error in"=w326, "PARAMETER/CONFIG"=TRUE, "Config Enum"=Config_file__FGV_Unitest_enum."READ") -> ("READ VALUE"=w327:string, "error out"=w331:errorcluster)  [unwired: 13 in]
  }
  n192 = Unbundle By Name("main ref") -> ("New PID LOGIC.PID SDelay"=w71:refnum<vi>)
  n193 = Unbundle By Name("main ref") -> ("New PID LOGIC.Kp"=w70:refnum<vi>)
  n194 = Unbundle By Name("main ref") -> ("New PID LOGIC.Ki"=w65:refnum<vi>)
  n195 = Unbundle By Name("main ref") -> ("New PID LOGIC.Kd"=w64:refnum<vi>)
  n196 = Unbundle By Name("main ref") -> ("New PID LOGIC.Deadband"=w60:refnum<vi>)
  n197 = Unbundle By Name("main ref") -> ("New PID LOGIC.pct_scale"=w59:refnum<vi>)
  n198 = Unbundle By Name("main ref") -> ("New PID LOGIC.Init Step"=w56:refnum<vi>)
  n199 = Unbundle By Name("main ref") -> ("New PID LOGIC.i_limit"=w55:refnum<vi>)
  n200 = Unbundle By Name("main ref") -> ("New PID LOGIC.Max Step Linit"=w52:refnum<vi>)
  n201 = Unbundle By Name("main ref") -> ("New PID LOGIC.Max_pos_limit"=w50:refnum<vi>)
  n202 = Unbundle By Name("main ref") -> ("New PID LOGIC.Min_pos_limit"=w49:refnum<vi>)
  n203 = Index Array(array=w47) -> (element #1=w46:string, element #2=w45:string, element #3=w42:string, element #4=w41:string, element #5=w40:string, element #6=w39:string, element #7=w34:string, element #8=w33:string, element #9=w32:string, element #10=w31:string, element #11=w30:string)  [unwired: 11 in]
  n204 = call "CONFIG FILE MAIN Unitest.vi"("error in"=w75, "Config Enum"=Config_file__FGV_Unitest_enum."CLOSE") -> ("error out"=→"error out":errorcluster)  [unwired: 16 in, 1 out]
  n205 = Fract/Exp String To Number(string=w46) -> (number=w44:dbl)  [unwired: 3 in, 1 out]
  n206 = Fract/Exp String To Number(string=w45) -> (number=w43:dbl)  [unwired: 3 in, 1 out]
  n207 = Fract/Exp String To Number(string=w42) -> (number=w38:dbl)  [unwired: 3 in, 1 out]
  n208 = Fract/Exp String To Number(string=w41) -> (number=w37:dbl)  [unwired: 3 in, 1 out]
  n209 = Fract/Exp String To Number(string=w40) -> (number=w36:dbl)  [unwired: 3 in, 1 out]
  n210 = Fract/Exp String To Number(string=w39) -> (number=w35:dbl)  [unwired: 3 in, 1 out]
  n211 = Fract/Exp String To Number(string=w34) -> (number=w29:dbl)  [unwired: 3 in, 1 out]
  n212 = Fract/Exp String To Number(string=w33) -> (number=w28:dbl)  [unwired: 3 in, 1 out]
  n213 = Fract/Exp String To Number(string=w32) -> (number=w27:dbl)  [unwired: 3 in, 1 out]
  n214 = Fract/Exp String To Number(string=w31) -> (number=w26:dbl)  [unwired: 3 in, 1 out]
  n215 = Fract/Exp String To Number(string=w30) -> (number=w25:dbl)  [unwired: 3 in, 1 out]
  n216 = property class="DigNum (strict)"(reference=w71, "Value"=w44) -> (reference out=w73:refnum<vi>, error out=w72:errorcluster)  [unwired: 1 in]
  n217 = property class="DigNum (strict)"(reference=w70, "Value"=w43) -> (reference out=w68:refnum<vi>, error out=w69:errorcluster)  [unwired: 1 in]
  n218 = property class="DigNum (strict)"(reference=w65, "Value"=w38) -> (reference out=w67:refnum<vi>, error out=w66:errorcluster)  [unwired: 1 in]
  n219 = property class="DigNum (strict)"(reference=w64, "Value"=w37) -> (reference out=w62:refnum<vi>, error out=w63:errorcluster)  [unwired: 1 in]
  n220 = property class="DigNum (strict)"(reference=w60, "Value"=w36) -> (reference out=w23:refnum<vi>, error out=w61:errorcluster)  [unwired: 1 in]
  n221 = property class="DigNum (strict)"(reference=w59, "Value"=w35) -> (reference out=w24:refnum<vi>, error out=w58:errorcluster)  [unwired: 1 in]
  n222 = property class="DigNum (strict)"(reference=w56, "Value"=w29) -> (reference out=w22:refnum<vi>, error out=w57:errorcluster)  [unwired: 1 in]
  n223 = property class="DigNum (strict)"(reference=w55, "Value"=w28) -> (reference out=w21:refnum<vi>, error out=w54:errorcluster)  [unwired: 1 in]
  n224 = property class="DigNum (strict)"(reference=w52, "Value"=w27) -> (reference out=w20:refnum<vi>, error out=w53:errorcluster)  [unwired: 1 in]
  n225 = property class="DigNum (strict)"(reference=w50, "Value"=w26) -> (reference out=w19:refnum<vi>, error out=w51:errorcluster)  [unwired: 1 in]
  n226 = property class="DigNum (strict)"(reference=w49, "Value"=w25) -> (reference out=w18:refnum<vi>, error out=w48:errorcluster)  [unwired: 1 in]
  n227 = Close Reference(reference=w73, error in (no error)=w72) -> ()  [unwired: 1 out]
  n228 = Close Reference(reference=w68, error in (no error)=w69) -> ()  [unwired: 1 out]
  n229 = Close Reference(reference=w67, error in (no error)=w66) -> ()  [unwired: 1 out]
  n230 = Close Reference(reference=w62, error in (no error)=w63) -> ()  [unwired: 1 out]
  n231 = Close Reference(reference=w23, error in (no error)=w61) -> ()  [unwired: 1 out]
  n232 = Close Reference(reference=w24, error in (no error)=w58) -> ()  [unwired: 1 out]
  n233 = Close Reference(reference=w22, error in (no error)=w57) -> ()  [unwired: 1 out]
  n234 = Close Reference(reference=w21, error in (no error)=w54) -> ()  [unwired: 1 out]
  n235 = Close Reference(reference=w20, error in (no error)=w53) -> ()  [unwired: 1 out]
  n236 = Close Reference(reference=w19, error in (no error)=w51) -> ()  [unwired: 1 out]
  n237 = Close Reference(reference=w18, error in (no error)=w48) -> ()  [unwired: 1 out]
